vi "usrp set rx lo source.vi"(7 "chan":u64, 8 "error in (no error)":errorcluster, 9 "name":string, 10 "src":string, 11 "h":u64) -> (0 "error out":errorcluster, 3 "function return":u32(ring))   [LabVIEW 2023, in "uhd.lvlib"]
doc: "UHD_API uhd_error uhd_usrp_set_rx_lo_source(\n uhd_usrp_handle h, const char* src, const char* name, size_t chan);"
uses:
  <userlib>/uhd/uhd.lvlib
  <userlib>/uhd/uhd.dll
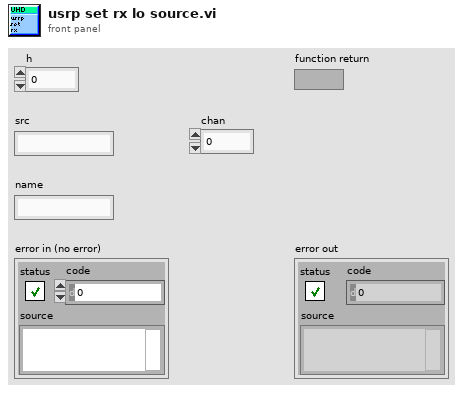
[diagram p1: front panel]
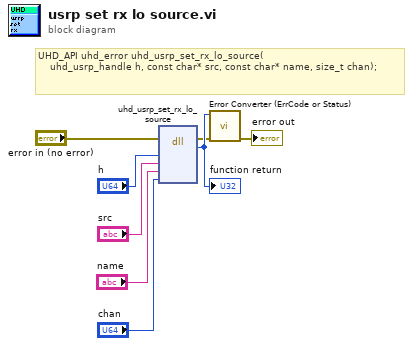
[diagram p0: block diagram]
diagram:
  # "UHD_API uhd_error uhd_usrp_set_rx_lo_source(\n    uhd_usrp_handle h, const char* src, const char* name, size_t chan);"
  n1 = dll-call lib="C:/Program Files/National Instruments/LabVIEW 2023/user.lib/uhd/uhd.*" fn="uhd_usrp_set_rx_lo_source"(error in="error in (no error)", "h"="h", "src"="src", "name"="name", "chan"="chan") -> (error out=w2:errorcluster, w8:u32)  [unwired: 6 in, 1 out]
  "function return" <- w8
  n2 = call <userlib>:"Error Converter (ErrCode or Status).vi"("error in (no error)"=w2, "error code"=w8) -> ("error out"=→"error out":errorcluster)  [unwired: 9 in]
